vi "ExposeMapperUdpateObject.vi"(8 "Allow Variant Values (f)":bool, 10 "Object Map":T1[](array[typedef]), 11 "Type (or value to update)":variant) -> (1 "Updated Controls":refnum<vi>[](array[refnum]), 3 "Value":variant)   [LabVIEW 2017]
uses:
  ExposeObjectMapNamepathData.ctl
  ExposeMapperDataTypeEnum.ctl
  ExposeObjectMapContainerTypeEnum.ctl
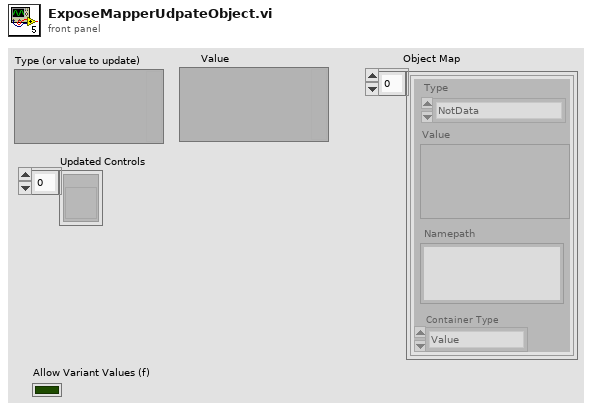
[diagram p1: front panel]
types:
  T1 = typedef "ExposeObjectMapNamepathData.ctl" = cluster{"Type":T2, "Value":variant, "Namepath":string, "Container Type":T3}
  T2 = typedef "ExposeMapperDataTypeEnum.ctl" = enum16{"NotData", "int8", "byte", "int16", "uint16", "int32", "uint32", "int64", "uint64", "Single", "Double", "String", "Boolean", "Container"}
  T3 = typedef "ExposeObjectMapContainerTypeEnum.ctl" = enum16{"Value", "Array", "Waveform", "NetContainer"}
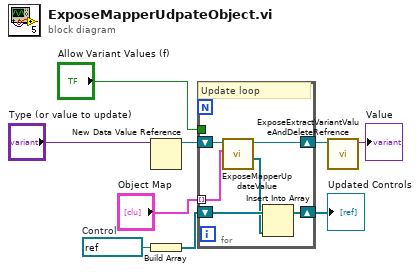
[diagram p0: block diagram]
diagram:
  w7 = refnum<vi> refnum  # Control
  n1 = New Data Value Reference(data value="Type (or value to update)") -> (data value reference=w3:refnum<data-value>)  [unwired: 1 in, 1 out]
  n2 = Build Array(w7) -> (w6:refnum<vi>[])
  n3 = for {
    tunnel: "Object Map" -> [w12] mode=indexing
    shift-right: [w11] -> w2
    shift-left: w3 -> [w13]
    tunnel: "Allow Variant Values (f)" -> [_]
    shift-right: [w14] -> w5
    shift-left: w6 -> [w15]
    # "Update loop"
    n4 = call "ExposeMapperUpdateValue.vi"("Namepath Info"=w12, "Value In (or type, reference)"=w13) -> ("Updated controls"=w10:refnum<vi>[], "Value Out Ref"=w11:refnum<data-value>)  [unwired: 8 in]
    n5 = Insert Into Array(array=w15, new element=w10) -> (w14:refnum<vi>[])  [unwired: 1 in]
  }
  "Updated Controls" <- w5
  n6 = call "ExposeExtractVariantValueAndDeleteRefrence.vi"("Data Value Reference in"=w2) -> ("Value out"=→"Value":variant)  [unwired: 10 in]
